vi "Measurements (Global).vi"() -> ()   [LabVIEW 2018]
panel:
  out "PCC Status":bool
  in  "Load I Meas":dbl[](array[numeric])
  in  "Load V Meas":dbl[](array[numeric])
  in  "Load Q Meas":dbl[](array[numeric])
  in  "Load P Meas":dbl[](array[numeric])
  in  "Gen I Meas":dbl[](array[numeric])
  in  "Gen V Meas":dbl[](array[numeric])
  in  "Gen Q Meas":dbl[](array[numeric])
  in  "Gen P Meas":dbl[](array[numeric])
  in  "PV I Meas":dbl[](array[numeric])
  in  "PV V Meas":dbl[](array[numeric])
  in  "PV Q Meas":dbl[](array[numeric])
  in  "PV P Meas":dbl[](array[numeric])
  in  "ES_2 I Meas":dbl[](array[numeric])
  in  "ES_2 V Meas":dbl[](array[numeric])
  in  "ES_1 I Meas":dbl[](array[numeric])
  in  "ES_1 V Meas":dbl[](array[numeric])
  in  "ES_2 Q Meas":dbl[](array[numeric])
  in  "ES_2 P Meas":dbl[](array[numeric])
  in  "ES_1 Q Meas":dbl[](array[numeric])
  in  "ES_1 P Meas":dbl[](array[numeric])
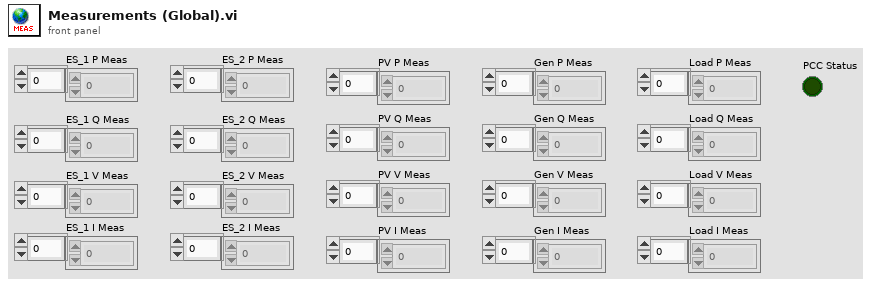
[diagram p1: front panel]
diagram:
